vi "T7_Read_UINT16_Register.vi"(6 "Num Registers to read":i32=2, 8 "error in (no error)":errorcluster, 9 "FirstChannel":i32, 10 "Remote Port":u16=502, 11 "Remote IP Address":string="192.168.126.148") -> (0 "error out":errorcluster, 1 "LastRead":timestamp=timestamp(3513857842.218402 s since 1904-01-01), 2 "Read UINT16":u16, 3 "Raw Data Read":u16[](array[numeric]))   [LabVIEW 2015]
uses:
  Serial Link Layer/NI_Modbus_Cleaned/NI Modbus121Clean.llb/MB Ethernet Master Query Read Input Registers (poly).vi
panel:
  out "Array":dbl[](array[numeric])
  out "LastValue":dbl
  # "MB Ethernet Example Master.vi\n\nInstructions\n1.Use Kipling to find your devices IP address & modify the\n\"Remote IP Addres\"\n2. Run this VI\n3. Change value of \"UINT16 to Write\" & press \"Write Data\""
  # "TCP Parameters"
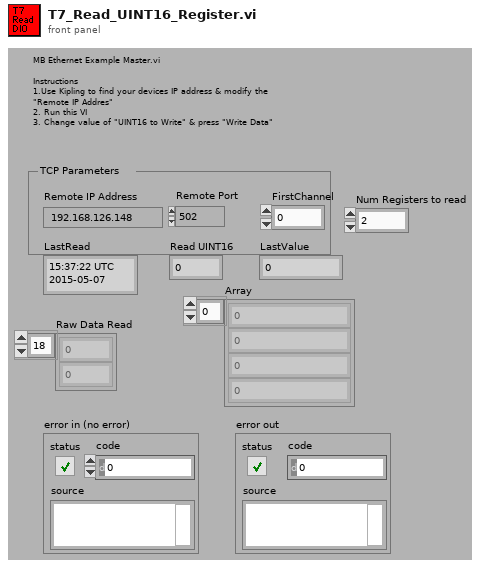
[diagram p1: front panel]
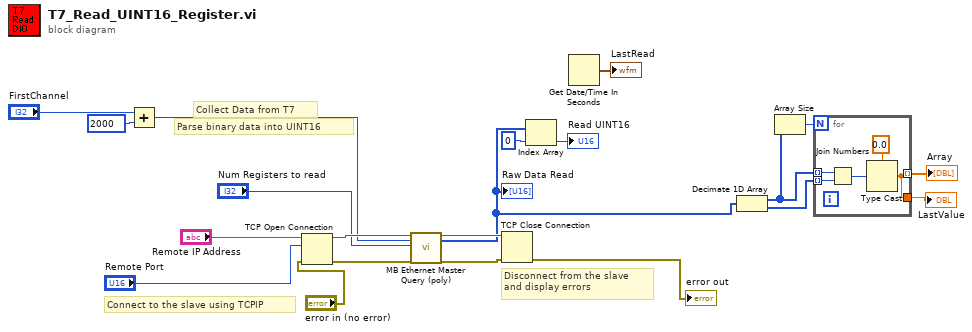
[diagram p0: block diagram]
diagram:
  # "Parse binary data into UINT16"
  # "Collect Data from T7"
  # "Disconnect from the slave\nand display errors"
  # "Connect to the slave using TCPIP"
  n1 = Add(x="FirstChannel", y=2000) -> (x+y=w11:i32)
  n2 = TCP Open Connection(address="Remote IP Address", remote port or service name="Remote Port", error in (no error)="error in (no error)") -> (connection ID=w19:refnum<k5>, error out=w18:errorcluster)  [unwired: 2 in]
  n3 = call-poly "MB Ethernet Master Query (poly).vi"("TCP Connection Refnum in"=w19, "Starting Address"=w11, "Quantity"="Num Registers to read", "error in"=w18) -> ("TCP Connection Refnum (dup)"=w16:refnum<k5>, "Input Registers"=w4:u16[], "error out"=w17:errorcluster)  [unwired: 12 in, 1 out]
  "Raw Data Read" <- w4
  n4 = TCP Close Connection(connection ID=w16, error in (no error)=w17) -> (error out=→"error out":errorcluster)  [unwired: 2 out]
  n5 = Index Array(array=w4, index=0) -> (element=→"Read UINT16":u16)
  n6 = Get Date/Time In Seconds() -> (seconds since 1Jan1904=→"LastRead":timestamp)
  n7 = Decimate 1D Array(w4) -> (w6:u16[], w7:u16[])
  n8 = Array Size(array=w6) -> (size(s)=w5:i32)
  n9 = for {
    N: w5 -> [_]
    tunnel: w6 -> [w25] mode=indexing
    tunnel: w7 -> [w26] mode=indexing
    tunnel: [w22] -> w8 mode=indexing
    tunnel: [w22] -> w9
    n10 = Join Numbers(hi=w25, lo=w26) -> ((hi.lo)=w24:u32)
    n11 = Type Cast(type=sgl 0.0, x=w24) -> (*(type *) &x=w22:sgl)
  }
  "Array" <- w8
  "LastValue" <- w9
